vi "5024_default_o_p_configure_.vi"() -> ()   [LabVIEW 2010]
uses:
  ADAM Client/Sub VIs/ADAM Controls/Address.ctl
panel:
  in  "Address (all reqd.)":T1={"Main"=0, "Ch."=0, "Sub"=0, "Port Name"="MainNetwork"}
  in  "Use checksum":bool
  out "Reply":string
  out "?":string
  # "Happy reply starts \"!\"\nUnhappy reply starts \"?\""
  # "Sets the default output to be the current output value"
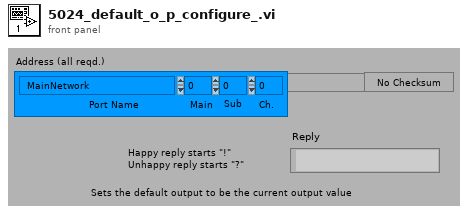
[diagram p1: front panel]
types:
  T1 = typedef "Address.ctl" = cluster{"Main":i32, "Ch.":i32, "Sub":i32, "Port Name":string}
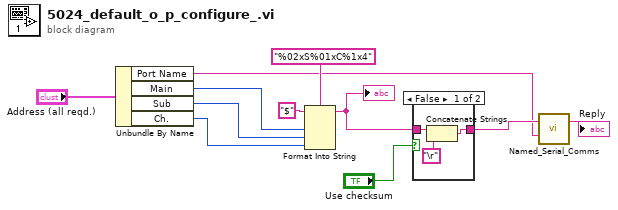
[diagram p0: block diagram]
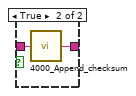
[diagram p2: hidden frame]
diagram:
  n1 = Unbundle By Name("Address (all reqd.)") -> ("Port Name"=w1:string, "Main"=w2:i32, "Sub"=w3:i32, "Ch."=w4:i32)
  n2 = Format Into String(format string="%02xS%01xC%1x4", initial string="$", w2, w3, w4) -> (resulting string=w9:string)  [unwired: 1 in, 1 out]
  "?" <- w9
  n3 = case shown="False" "Use checksum" {
    tunnel: w9 -> [w14 w16]
    tunnel: [w13 w15] -> w7
    frame False {
      n4 = Concatenate Strings(w14, "\r") -> (w13:string)
    }
    frame True {
      n5 = call "4000_Append_checksum.vi"("ADAM command"=w16) -> ("ADAM string to send"=w15:string)
    }
  }
  n6 = call "Named_Serial_Comms.vi"("Write String"=w7, "Port Name"=w1) -> ("Read"=→"Reply":string)  [unwired: 10 in, 3 out]
